vi "BasicTrigEdge.vi"(0 "task out 2":refnum<k24>, 1 "error out 2":errorcluster) -> (2 "task out":refnum<k24>, 3 "Edge":i32(ring) items=["Rising", "Falling"], 4 "error out":errorcluster)   [LabVIEW 2009]
uses:
  C:/Program Files/National Instruments/LabVIEW 2009/vi.lib/ULx/ULx_LV.dll
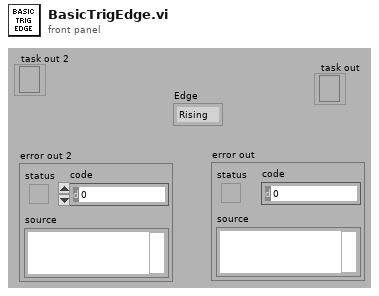
[diagram p1: front panel]
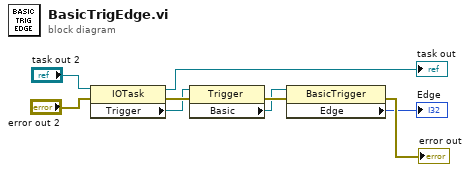
[diagram p0: block diagram]
diagram:
  n1 = property class="IOTask"(reference="task out 2", error in="error out 2") -> (reference out=→"task out":refnum<k24>, error out=w7:errorcluster, "Trigger"=w4:refnum<k24>)
  n2 = property class="Trigger"(reference=w4, error in=w7) -> (error out=w8:errorcluster, "Basic"=w5:refnum<k24>)  [unwired: 1 out]
  n3 = property class="BasicTrigger"(reference=w5, error in=w8) -> (error out=→"error out":errorcluster, "Edge"=→"Edge":i32)  [unwired: 1 out]
